vi "S2C_FORNAX_Proc_ViperMsgScan.vi"(8 "Error In":errorcluster, 11 "Message":string) -> (0 "Error Out":errorcluster)   [LabVIEW 2015]
doc: "Extracts the Viper message from the DDS data stream."
uses:
  S2C_FORNAX_Proc_Globals.vi
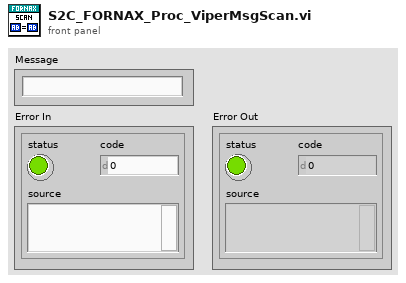
[diagram p1: front panel]
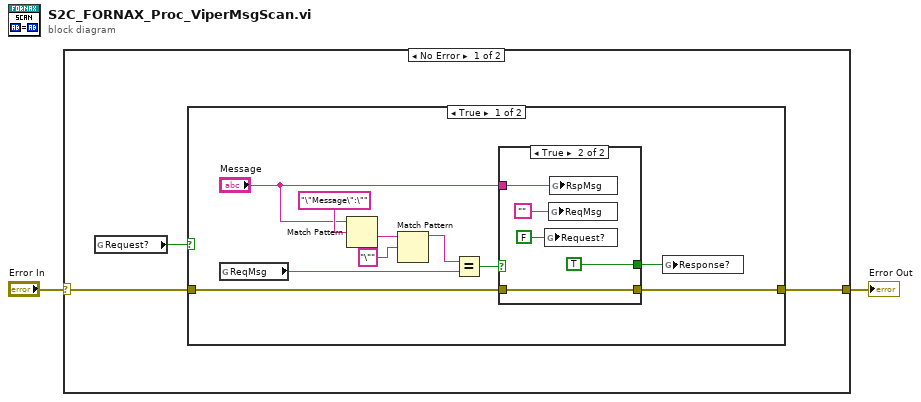
[diagram p0: block diagram]
diagram:
  n1 = case shown="No Error" "Error In" {
    selector: "Error In" -> [w5 w23]
    tunnel: [w4 w23] -> w1
    frame No Error {
      n2 = global read "S2C_FORNAX_Proc_Globals.vi" "Request?"() -> (w3:bool)
      n3 = case shown="True" w3 {
        tunnel: w5 -> [w11 w22]
        tunnel: [w9 w22] -> w4
        frame True {
          n4 = global read "S2C_FORNAX_Proc_Globals.vi" "ReqMsg"() -> (w8:string)
          n5 = Match Pattern(string="Message", regular expression="\"Message\":\"") -> (after substring=w14:string)  [unwired: 1 in, 3 out]
          n6 = Match Pattern(string=w14, regular expression="\"") -> (before substring=w12:string)  [unwired: 1 in, 3 out]
          n7 = Equal?(x=w12, y=w8) -> (x = y?=w10:bool)
          n8 = case shown="True" w10 {
            tunnel: w11 -> [w16 w19]
            tunnel: "Message" -> [_ w21]
            tunnel: [w16 w19] -> w9
            tunnel: [_ TRUE] -> w7
            frame False {
            }
            frame True {
              n9 = global write "S2C_FORNAX_Proc_Globals.vi" "Request?"(FALSE) -> ()
              n10 = global write "S2C_FORNAX_Proc_Globals.vi" "ReqMsg"("") -> ()
              n11 = global write "S2C_FORNAX_Proc_Globals.vi" "RspMsg"(w21) -> ()
            }
          }
          n12 = global write "S2C_FORNAX_Proc_Globals.vi" "Response?"(w7) -> ()
        }
        frame False {
        }
      }
    }
    frame Error {
    }
  }
  "Error Out" <- w1
